vi "Close.vi"(8 "error in (no error)":errorcluster, 11 "Yokogawa WT500 in":refnum<class "Yokogawa WT500.lvclass">) -> (0 "error out":errorcluster, 3 "Yokogawa WT500 out":refnum<class "Yokogawa WT500.lvclass">)   [LabVIEW 2016, in "Generic Power Analyzer.lvlib" / "Yokogawa WT500.lvlib" / "Yokogawa WT500.lvclass"]
uses:
  Yokogawa WT500.lvclass
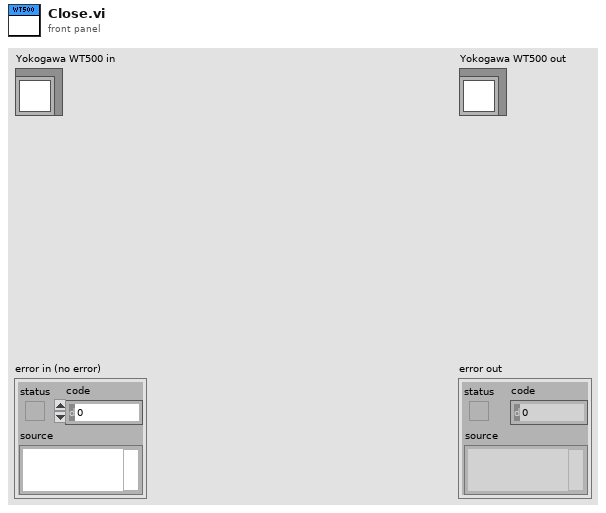
[diagram p1: front panel]
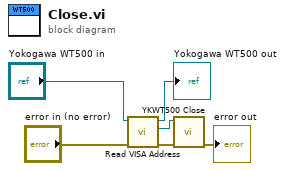
[diagram p0: block diagram]
diagram:
  n1 = call-dynamic "Read VISA Address.vi"("error in (no error)"="error in (no error)", "Generic Device in"="Yokogawa WT500 in") -> ("error out"=w3:errorcluster, "VISA Address"=w2:refnum<visa-resource-name>, "Generic Device out"=→"Yokogawa WT500 out":refnum<class "Yokogawa WT500.lvclass">)  [unwired: 7 in]
  n2 = call <instrlib>:"YKWT500 Close.vi"("error in (no error)"=w3, "VISA resource name"=w2) -> ("error out"=→"error out":errorcluster)  [unwired: 9 in]
